vi "Update Tree.vi"(7 "Filter":T1, 8 "error in (no error)":errorcluster, 9 "Test Tree":refnum<vi>, 10 "Result Model":refnum<class "Result Model.lvclass">) -> (0 "error out":errorcluster)   [LabVIEW 2020, in "Test Result View.lvlib" / "Test Result View.lvclass"]
uses:
  Test Result View.lvclass
  Test Result View.lvclass/Test Result View.ctl
  User Interface/Result Model/Result Model.lvclass
  User Interface/Result Model/Tree Item Filter.ctl
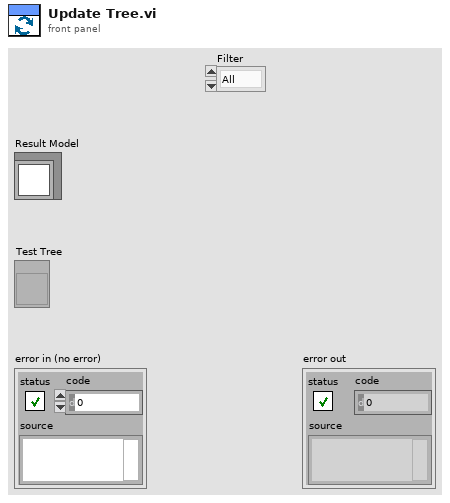
[diagram p1: front panel]
types:
  T1 = typedef "Result Model.lvclass/Tree Item Filter.ctl" = enum16{"All", "Only Fails"}
  T2 = cluster{"Left Cell String":string, "Child Text":string[], "Child Tag":string, "Item Indent":i32, "Child Only?":bool, "Glyph Index":i32}[]
  T3 = typedef "LVNodeAndColumnTypeDef.ctl" = cluster{"Node":string, "Column":i32}
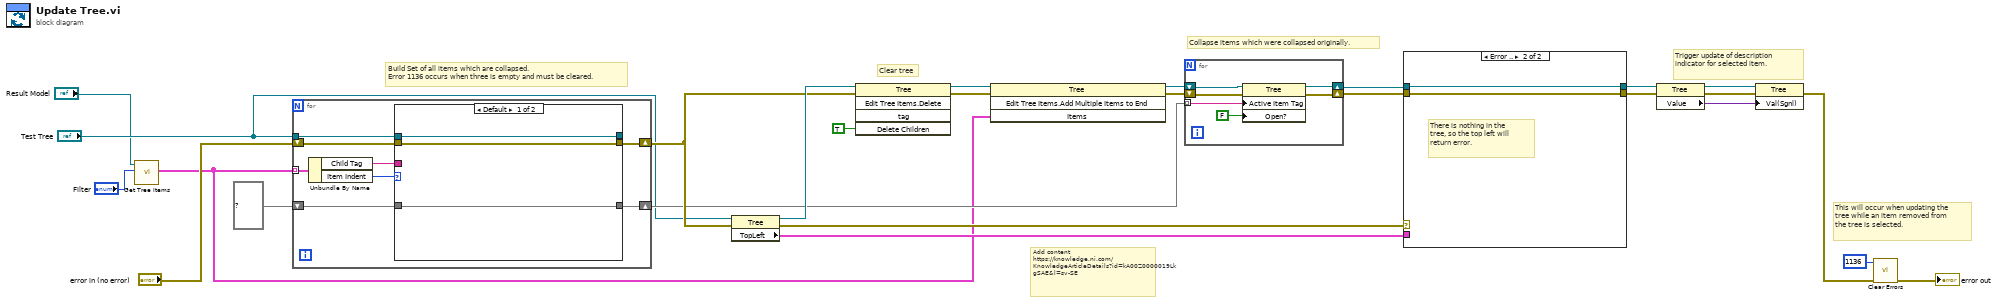
[diagram p0: block diagram]
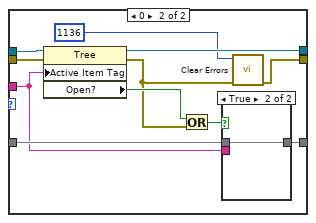
[diagram p2: hidden frame]
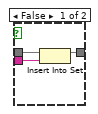
[diagram p3: hidden frame]
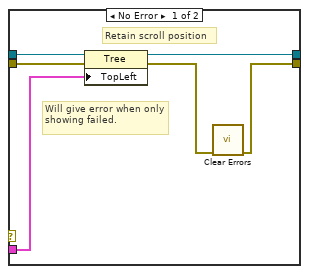
[diagram p4: hidden frame]
diagram:
  # "Collapse items which were collapsed originally."
  # "Build Set of all items which are collapsed.\nError 1136 occurs when three is empty and must be cleared."
  # "This will occur when updating the tree while an item removed from the tree is selected."
  # "Trigger update of description indicator for selected item."
  # "Add content\nhttps://knowledge.ni.com/KnowledgeArticleDetails?id=kA00Z0000019LkgSAE&l=sv-SE"
  # "Clear tree"
  n1 = call "Get Tree Items.vi"("Filter"="Filter", "Result Model In"="Result Model") -> ("Tree Items"=w4:T2)  [unwired: 8 in, 1 out]
  n2 = for {
    tunnel: w4 -> [w34] mode=indexing
    shift-right: [w28] -> w13
    shift-left: "error in (no error)" -> [w29]
    shift-right: [w31] -> w11
    shift-left: set{string} {} ("set") -> [w32]
    tunnel: "Test Tree" -> [w33]
    n3 = Unbundle By Name(w34) -> ("Child Tag"=w30:string, "Item Indent"=w27:i32)
    n4 = case shown="Default" w27 {
      tunnel: w33 -> [w36 w48]
      tunnel: [w36 w47] -> _
      tunnel: w32 -> [w37 w46]
      tunnel: [w37 w45] -> w31
      tunnel: w30 -> [_ w44]
      tunnel: w29 -> [w35 w42]
      tunnel: [w35 w41] -> w28
      frame Default {
      }
      frame 0 {
        n5 = property class="Tree"(reference=w48, error in=w42, "Active Item Tag"=w44) -> (reference out=w47:refnum<vi>, error out=w38:errorcluster, "Open?"=w43:bool)
        n6 = Or(x=w43, y=w38) -> (x .or. y?=w39:bool)
        n7 = case shown="True" w39 {
          tunnel: w46 -> [w51 w52]
          tunnel: [w50 w52] -> w45
          tunnel: w44 -> [w49 _]
          frame False {
            n8 = Insert Into Set(10:w49, 11:w51) -> (3:w50:set{string})  [unwired: 1 out]
          }
          frame True {
          }
        }
        n9 = call <vilib>:"Clear Errors.vi"("error in (no error)"=w38, "specific error code to clear (0: all)"=1136) -> ("error out"=w41:errorcluster)  [unwired: 4 in, 1 out]
      }
    }
  }
  n10 = property on="Property Node" class="Tree"(reference="Test Tree", error in=w13) -> (reference out=w23:refnum<vi>, error out=w22:errorcluster, "TopLeft"=w21:T3)
  n11 = invoke on="Invoke Node" class="Tree" method="Edit Tree Items.Delete"(reference=w23, error in=w13, "Delete Children"=TRUE ("Delete Children?")) -> (reference out=w25:refnum<vi>, error out=w24:errorcluster)  [unwired: 2 in, 3 out]
  n12 = invoke class="Tree" method="Edit Tree Items.Add Multiple Items to End"(reference=w25, error in=w24, "Items"=w4) -> (reference out=w8:refnum<vi>, error out=w5:errorcluster)  [unwired: 1 in, 2 out]
  n13 = for {
    shift-right: [w57] -> w7
    shift-left: w8 -> [w58]
    shift-right: [w56] -> w6
    shift-left: w5 -> [w55]
    tunnel: w11 -> [w54] mode=indexing
    n14 = property class="Tree"(reference=w58, error in=w55, "Active Item Tag"=w54, "Open?"=FALSE ("Active Item:Open?")) -> (reference out=w57:refnum<vi>, error out=w56:errorcluster)
  }
  n15 = case shown="Error .." w22 {
    tunnel: w7 -> [w64 w66]
    tunnel: [w63 w66] -> w10
    tunnel: w6 -> [w62 w65]
    tunnel: [w59 w65] -> w9
    tunnel: w21 -> [w60 _]
    frame No Error {
      # "Will give error when only showing failed."
      # "Retain scroll position"
      n16 = property on="Property Node" class="Tree"(reference=w64, error in=w62, "TopLeft"=w60) -> (reference out=w63:refnum<vi>, error out=w61:errorcluster)
      n17 = call <vilib>:"Clear Errors.vi"("error in (no error)"=w61) -> ("error out"=w59:errorcluster)  [unwired: 5 in, 1 out]
    }
    frame Error {
      # "There is nothing in the tree, so the top left will return error."
    }
  }
  n18 = property on="Property Node" class="Tree"(reference=w10, error in=w9) -> (reference out=w20:refnum<vi>, error out=w19:errorcluster, "Value"=w17:variant)
  n19 = property on="Property Node" class="Tree"(reference=w20, error in=w19, "Val(Sgnl)"=w17) -> (error out=w18:errorcluster)  [unwired: 1 out]
  n20 = call <vilib>:"Clear Errors.vi"("error in (no error)"=w18, "specific error code to clear (0: all)"=1136) -> ("error out"=→"error out":errorcluster)  [unwired: 4 in, 1 out]
